vi "Workspace.ConnectionPath.Create.vi"(10 "Bus":enum16{"Primary Bus", "Ghost Bus"}(ring), 11 "Addon Name":string) -> (3 "Connection Path":string)   [LabVIEW 2019, in "Ghost Bus Workspace Shared.lvlib"]
uses:
  Ghost Bus Workspace Shared.lvlib
  Addon/Addon Shared/SubVIs/GUID Lookup.vi
  Addon/Addon Shared/Ghost Bus Addon Shared.lvlib
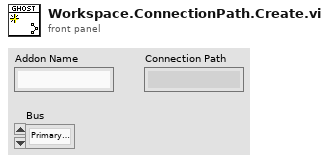
[diagram p1: front panel]
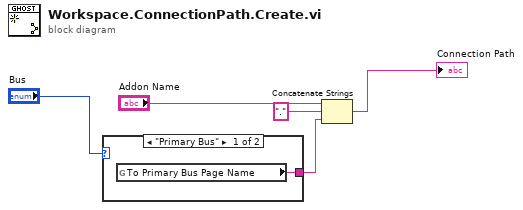
[diagram p0: block diagram]
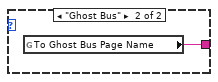
[diagram p2: hidden frame]
diagram:
  n1 = case shown="\"Primary Bus\"" "Bus" {
    tunnel: [w6 w7] -> w3
    frame "Primary Bus" {
      n2 = global read "GUID Lookup.vi" "To Primary Bus Page Name"() -> (w6:string)
    }
    frame "Ghost Bus" {
      n3 = global read "GUID Lookup.vi" "To Ghost Bus Page Name"() -> (w7:string)
    }
  }
  n4 = Concatenate Strings("Addon Name", "." ("string"), w3) -> (→"Connection Path":string)
